vi "Update Parameter.vi"(8 "error in":errorcluster, 9 "parameter definition":T1, 10 "data":dbl, 11 "32-bit Word in":refnum<class "32-bit Word.lvclass">) -> (0 "error out":errorcluster, 1 "signed?":bool, 3 "32-bit Word out":refnum<class "32-bit Word.lvclass">)   [LabVIEW 2020, in "32-bit Word.lvclass"]
uses:
  32-bit Word.lvclass
  Parameter Definition.ctl
  <vilib>/NI/NI VeriStand Encoding and Decoding/Encoding.ctl
  32-bit Word.lvclass/32-bit Word.ctl
  Read 32-Bit Word.vi
  Write 32-Bit Word.vi
  <vilib>/NI/NI VeriStand Encoding and Decoding/Encoding and Decoding.lvlib
  ARINC 429.lvclass
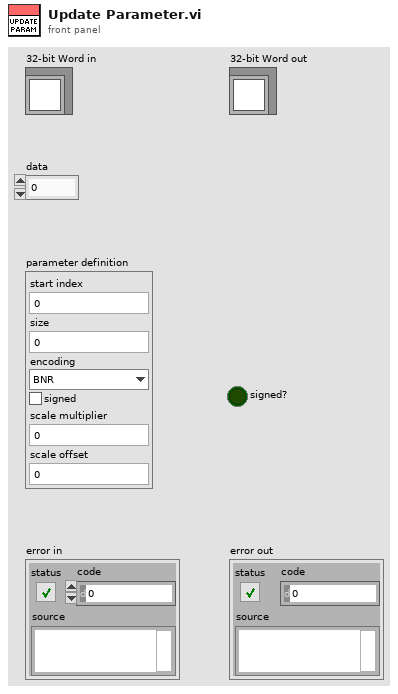
[diagram p1: front panel]
types:
  T1 = typedef "ARINC 429.lvclass/Parameter Definition.ctl" = cluster{"start index":i32, "size":i32, "encoding":T2, "signed":bool, "scale multiplier":dbl, "scale offset":dbl}
  T2 = typedef "Encoding and Decoding.lvlib/Encoding.ctl" = enum16{"BNR", "BCD", "Discrete"}
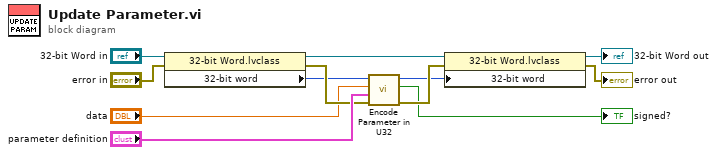
[diagram p0: block diagram]
diagram:
  n1 = property on="Property Node" class="32-bit Word.lvclass"(reference="32-bit Word in", error in="error in") -> (reference out=w3:refnum<class "32-bit Word.lvclass">, error out=w10:errorcluster, "32-bit word"=w2:u32)
  n2 = call "Encode Parameter in U32.vi"("error in"=w10, "parameter definition"="parameter definition", "data"="data", "32-bit word in"=w2) -> ("error out"=w11:errorcluster, "signed?"=→"signed?":bool, "32-bit word out"=w5:u32)  [unwired: 5 in]
  n3 = property on="Property Node" class="32-bit Word.lvclass"(reference=w3, error in=w11, "32-bit word"=w5) -> (reference out=→"32-bit Word out":refnum<class "32-bit Word.lvclass">, error out=→"error out":errorcluster)
